vi "configReset.vi"(7 "address":string, 8 "error in (no error)":errorcluster, 10 "Reset":bool=TRUE) -> (0 "error out":errorcluster)   [LabVIEW 2016]
doc: "API to put lockin into remote mode.\n\nIf address=\"\", this API reads from localhost\nIf address is remote lockin, you need to add this computer to allowed whitelist on the lockin computer you are trying to access."
uses:
  Instrument.Lockin/Typedefs/Instrument.Lockin.Commands--Enum.ctl
  RemoteControl/LockinRemoteControl.lvclass
  Instrument.Lockin/Instrument.Lockin.lvclass
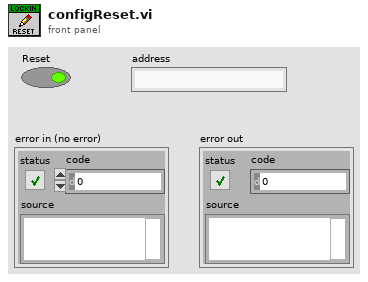
[diagram p1: front panel]
types:
  T1 = typedef "Instrument.Lockin.lvclass/Instrument.Lockin.Commands--Enum.ctl" = enum16{"configAO", "configREF", "configREFfilter", "configIVmode", "configRemote", "configReset", "configSampling", "assertTrigger", "getAO", "getAI", "getResults", "getTrigger", "getIVmode", "getSampling", "getAOconfig", "getREFconfig", "getREFfilter", "ACK", "UNK", "CLOSE", "configGain", "getGain"}
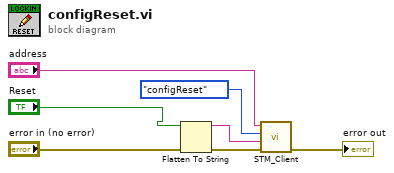
[diagram p0: block diagram]
diagram:
  n1 = Flatten To String(anything="Reset", error in (no error)="error in (no error)") -> (data string=w2:string, error out=w3:errorcluster)  [unwired: 2 in, 1 out]
  n2 = call "STM_Client.vi"("error in (no error)"=w3, "data to send"=w2, "Command"=Instrument.Lockin.Commands--Enum."configReset", "address"="address") -> ("error out"=→"error out":errorcluster)  [unwired: 6 in, 1 out]
